vi "testGetEnumSummaryState.vi"(8 "error in (no error)":errorcluster) -> (0 "error out":errorcluster)   [LabVIEW 2018]
uses:
  src/SalProcess/SalProcess.lvclass
  src/TypeDef/summaryState.ctl
  <vilib>/addons/_JKI Toolkits/Caraya/classes/Assert/Assert Equal Value and Type_Variant.vi
  <vilib>/addons/_JKI Toolkits/Caraya/classes/Test/Test.lvclass
  <vilib>/addons/_JKI Toolkits/Caraya/classes/Assert/Assert.lvclass
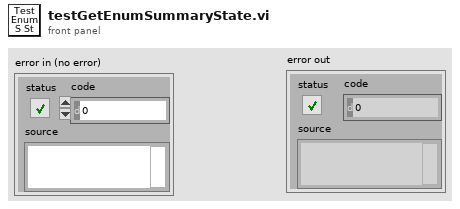
[diagram p1: front panel]
types:
  T1 = typedef "summaryState.ctl" = enum16{"", "DisabledState", "EnabledState", "FaultState", "OfflineState", "StandbyState"}
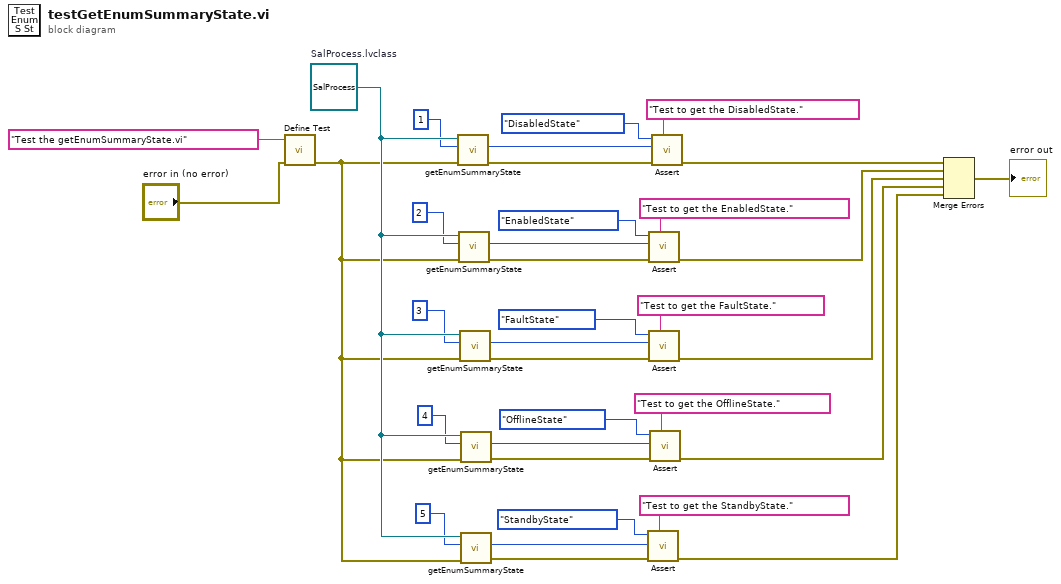
[diagram p0: block diagram]
diagram:
  w33 = refnum<class "SalProcess.lvclass"> refnum  # SalProcess.lvclass
  n1 = call <vilib>:"Define Test.vi"("error in (no error)"="error in (no error)", "Label (VI Title)"="Test the getEnumSummaryState.vi") -> ("error out"=w30:errorcluster)  [unwired: 9 in]
  n2 = call "getEnumSummaryState.vi"("error in (no error)"=w30, "valSummaryState"=1, "SalProcess in"=w33) -> ("error out"=w26:errorcluster, "enumSummaryState"=w25:T1)  [unwired: 6 in, 1 out]
  n3 = call "getEnumSummaryState.vi"("error in (no error)"=w30, "valSummaryState"=2, "SalProcess in"=w33) -> ("error out"=w18:errorcluster, "enumSummaryState"=w19:T1)  [unwired: 6 in, 1 out]
  n4 = call "getEnumSummaryState.vi"("error in (no error)"=w30, "valSummaryState"=3, "SalProcess in"=w33) -> ("error out"=w16:errorcluster, "enumSummaryState"=w17:T1)  [unwired: 6 in, 1 out]
  n5 = call "getEnumSummaryState.vi"("error in (no error)"=w30, "valSummaryState"=4, "SalProcess in"=w33) -> ("error out"=w14:errorcluster, "enumSummaryState"=w15:T1)  [unwired: 6 in, 1 out]
  n6 = call "getEnumSummaryState.vi"("error in (no error)"=w30, "valSummaryState"=5, "SalProcess in"=w33) -> ("error out"=w12:errorcluster, "enumSummaryState"=w13:T1)  [unwired: 6 in, 1 out]
  n7 = call-poly <vilib>:"Assert.vi"("Label"="Test to get the StandbyState.", "error in (no error)"=w12, "Y"=w13, "X"=summaryState."StandbyState" ("summaryState")) -> ("error out"=w2:errorcluster)  [unwired: 7 in]
  n8 = call-poly <vilib>:"Assert.vi"("Label"="Test to get the EnabledState.", "error in (no error)"=w18, "Y"=w19, "X"=summaryState."EnabledState" ("summaryState")) -> ("error out"=w5:errorcluster)  [unwired: 7 in]
  n9 = call-poly <vilib>:"Assert.vi"("Label"="Test to get the FaultState.", "error in (no error)"=w16, "Y"=w17, "X"=summaryState."FaultState" ("summaryState")) -> ("error out"=w4:errorcluster)  [unwired: 7 in]
  n10 = call-poly <vilib>:"Assert.vi"("Label"="Test to get the OfflineState.", "error in (no error)"=w14, "Y"=w15, "X"=summaryState."OfflineState" ("summaryState")) -> ("error out"=w3:errorcluster)  [unwired: 7 in]
  n11 = call-poly <vilib>:"Assert.vi"("Label"="Test to get the DisabledState.", "error in (no error)"=w26, "Y"=w25, "X"=summaryState."DisabledState" ("summaryState")) -> ("error out"=w6:errorcluster)  [unwired: 7 in]
  n12 = Merge Errors(w6, w5, w4, w3, w2) -> (→"error out":errorcluster)
